vi "Find Setpoints in Dictionary.vi"(8 "error in (no error)":errorcluster, 9 "processing data dictionary":refnum<class "data dictionary.lvclass">, 10 "PID Channels In":T1(array[cluster]), 11 "Tagbus PID Module runtime":refnum<class "Tagbus PID Module runtime.lvclass">) -> (0 "error out":errorcluster, 3 "Tagbus PID Module output":refnum<class "Tagbus PID Module runtime.lvclass">)   [LabVIEW 2014, in "Tagbus PID Module runtime.lvclass"]
uses:
  Tagbus PID Module runtime.lvclass
  <vilib>/NI/Tag Bus/dictionary/data dictionary.lvclass
  <vilib>/NI/Tag Bus Module Framework/channel/TBM channel.lvclass
  <vilib>/NI/Tag Bus/tag/Data Type.ctl
  Tagbus PID Module runtime.lvclass/Tagbus PID Module runtime.ctl
  <vilib>/NI/Tag Bus/tag/tag descriptor.lvclass
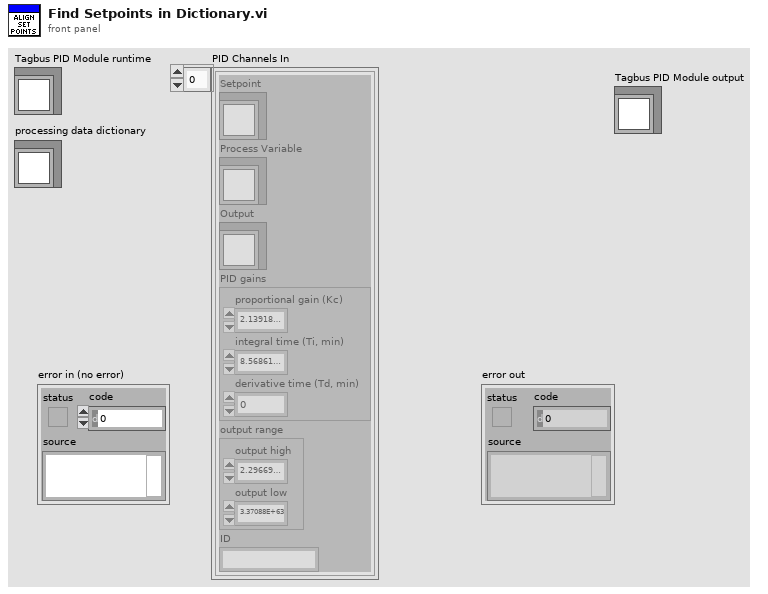
[diagram p1: front panel]
types:
  T1 = cluster{"Setpoint":refnum<class "TBM channel.lvclass">, "Process Variable":refnum<class "TBM channel.lvclass">, "Output":refnum<class "TBM channel.lvclass">, "PID gains":cluster{"proportional gain (Kc)":dbl, "integral time (Ti, min)":dbl, "derivative time (Td, min)":dbl}, "output range":cluster{"output high":dbl, "output low":dbl}, "ID":string}[]
  T2 = typedef "tag bus.lvlib/tag descriptor.lvclass/Data Type.ctl" = enum16{"Double", "Single", "I64", "I32", "I16", "I8", "U64", "U32", "U16", "U8", "Boolean", "String", "Array of Double", "Array of Single", "Array of I64", "Array of I32", "Array of I16", "Array of I8", "Array of U64", "Array of U32", "Array of U16", "Array of U8", "Array of Boolean", "Array of String"}
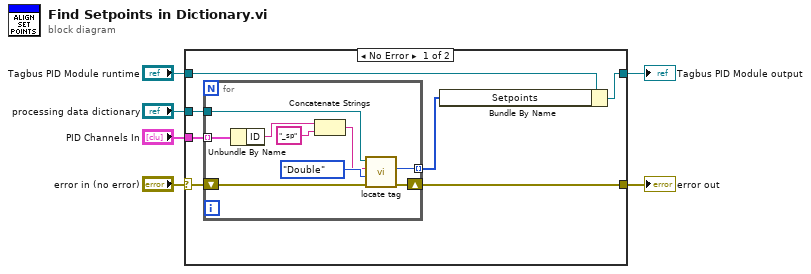
[diagram p0: block diagram]
diagram:
  n1 = case shown="No Error" "error in (no error)" {
    selector: "error in (no error)" -> [w11 w24]
    tunnel: [w10 w24] -> w5
    tunnel: "processing data dictionary" -> [w13 _]
    tunnel: "PID Channels In" -> [w12 _]
    tunnel: "Tagbus PID Module runtime" -> [w9 w23]
    tunnel: [w7 w23] -> w1
    frame No Error {
      n2 = for {
        tunnel: w13 -> [w21]
        tunnel: w12 -> [w22] mode=indexing
        shift-right: [w18] -> w10
        shift-left: w11 -> [w19]
        tunnel: [w17] -> w8 mode=indexing
        n3 = Unbundle By Name(w22) -> ("ID"=w16:string)
        n4 = Concatenate Strings(w16, "_sp" ("string")) -> (w14:string)
        n5 = call <vilib>:"locate tag.vi"("error in"=w19, "data type"=Data_Type."Double", "name"=w14, "data dictionary in"=w21) -> ("error out"=w18:errorcluster, "index"=w17:i32)  [unwired: 5 in, 1 out]
      }
      n6 = Bundle By Name(cluster=w9, "Setpoints"=w8) -> (w7:refnum<class "Tagbus PID Module runtime.lvclass">)
    }
    frame Error {
    }
  }
  "error out" <- w5
  "Tagbus PID Module output" <- w1
